vi "write galvo tasks.vi"(8 "error in (no error)":errorcluster, 11 "Waveform in":refnum<class "Waveform.lvclass">) -> (0 "error out":errorcluster, 3 "Waveform out":refnum<class "Waveform.lvclass">)   [LabVIEW 2012, in "Waveform.lvclass"]
uses:
  Waveform.lvclass
  Waveform.lvclass/Waveform.ctl
  <vilib>/DAQmx/write.llb/DAQmx Write (Analog Wfm 1Chan NSamp).vi
  <vilib>/DAQmx/miscellaneous.llb/DAQmx Fill In Error Info.vi
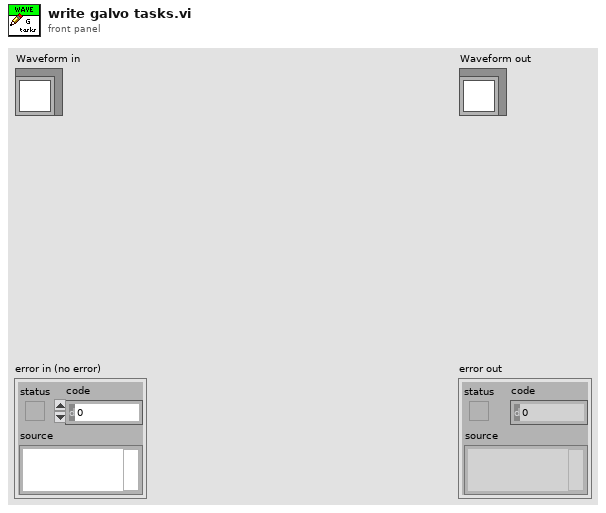
[diagram p1: front panel]
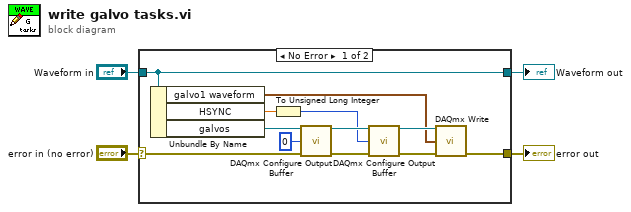
[diagram p0: block diagram]
diagram:
  n1 = case shown="No Error" "error in (no error)" {
    selector: "error in (no error)" -> [w7 w18]
    tunnel: [w15 w18] -> w3
    tunnel: [w16 w17] -> w1
    tunnel: "Waveform in" -> [w16 w17]
    frame No Error {
      n2 = Unbundle By Name(w16) -> ("galvo1 waveform"=w5:waveform(dbl), "HSYNC"=w11:dbl, "galvos"=w6:refnum<k21>)
      n3 = To Unsigned Long Integer(number=w11) -> (unsigned 32bit integer=w8:u32)
      n4 = call <vilib>:"DAQmx Configure Output Buffer.vi"("task/channels in"=w6, "buffer size (in samples per channel)"=u32 0, "error in"=w7) -> ("task out"=w9:refnum<k21>, "error out"=w13:errorcluster)  [unwired: 11 in]
      n5 = call <vilib>:"DAQmx Configure Output Buffer.vi"("task/channels in"=w9, "buffer size (in samples per channel)"=w8, "error in"=w13) -> ("task out"=w10:refnum<k21>, "error out"=w12:errorcluster)  [unwired: 11 in]
      n6 = call-poly <vilib>:"DAQmx Write.vi"("task/channels in"=w10, "data"=w5, "error in"=w12) -> ("error out"=w15:errorcluster)  [unwired: 10 in, 2 out]
    }
    frame Error {
    }
  }
  "error out" <- w3
  "Waveform out" <- w1
